vi "Main_Console.vi"(0 "Value_In":string="0" caption="Value In", 5 "Command":T1(ring), 7 "Log_File_Folder":path=path "D:/Assignments/Assignment-4/Assignment-4.1/Assignment-4.1-LV21V/CSV/Logger.csv" caption="Log File Folder", 9 "Stop":bool) -> (4 "Value_Out":string caption="Value Out")   [LabVIEW 2021]
doc: "This VI is the Console VI which communicate with Sour_Meas_instrument."
uses:
  <vilib>/Utility/file.llb/Write Delimited Spreadsheet (string).vi
panel:
  out "Error_Out":errorcluster
  in  "Error_In":errorcluster
  # "Control"
  # "Display"
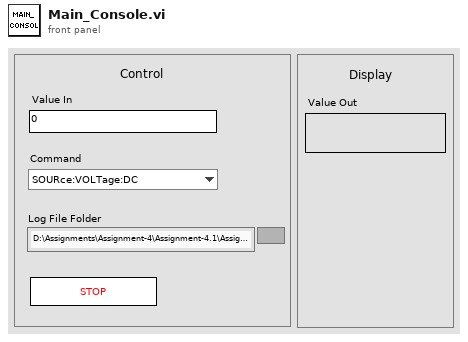
[diagram p1: front panel]
types:
  T1 = enum16{"SOURce:VOLTage:DC", "SOURce:CURRent:DC", "MEASure:VOLTage:DC?", "MEASure:CURRent:DC?"}
  T2 = enum16{"Left Button", "Center Button", "Right Button", "Window Close"}
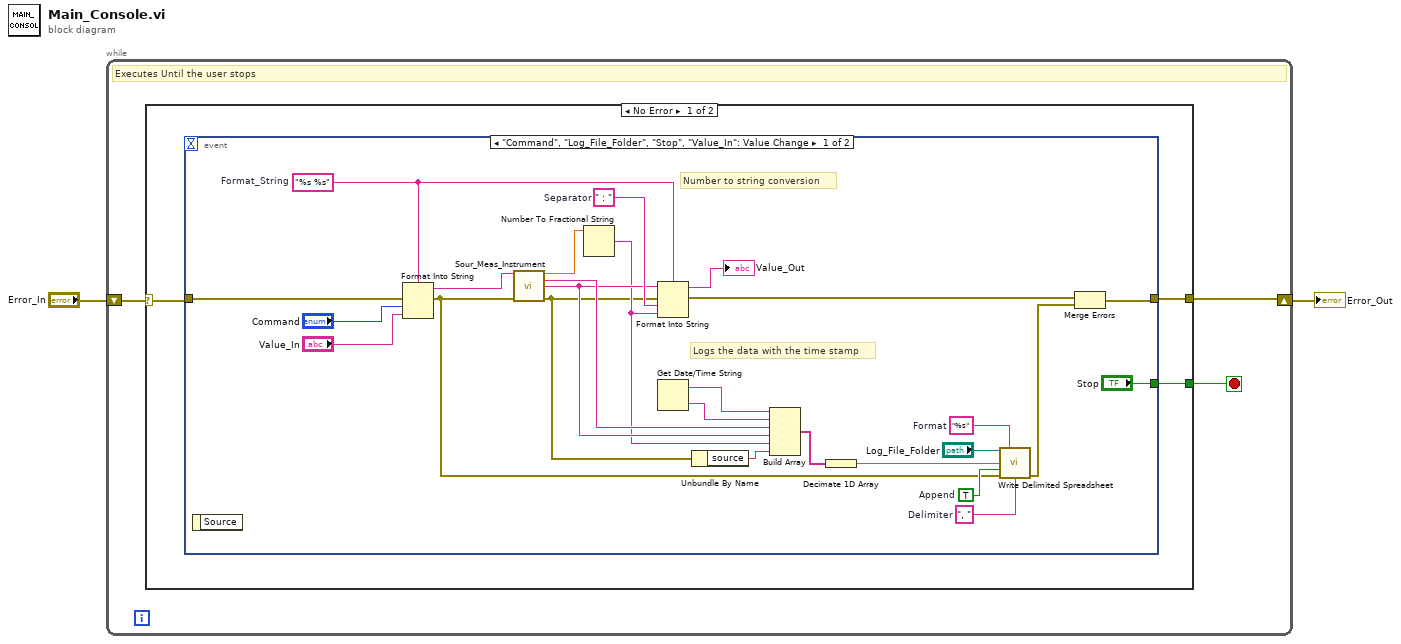
[diagram p0: block diagram]
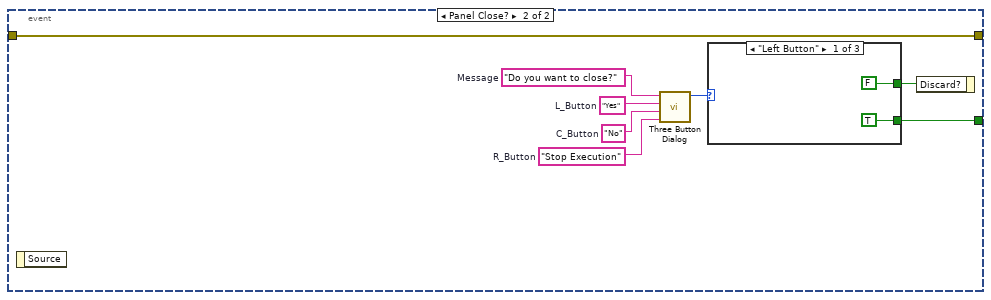
[diagram p2: hidden frame]
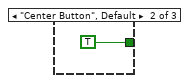
[diagram p3: hidden frame]
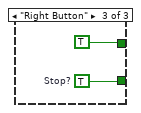
[diagram p4: hidden frame]
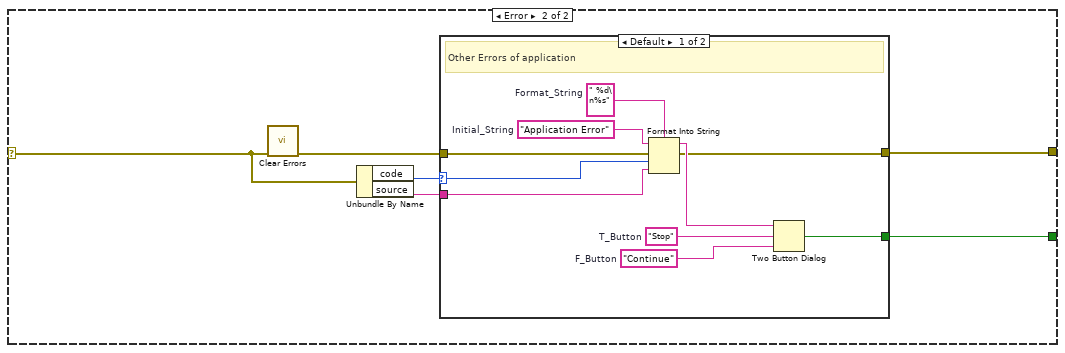
[diagram p5: hidden frame]
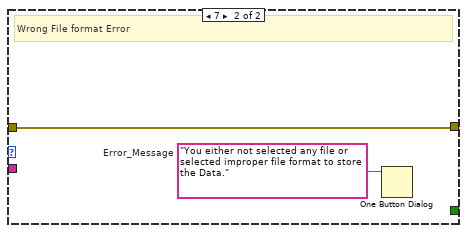
[diagram p6: hidden frame]
diagram:
  n1 = while {
    shift-right: [w3] -> w2
    shift-left: "Error_In" -> [w4]
    stop <- w5 stop-if-true
    # "Executes Until the user stops"
    n2 = case shown="No Error" w4 {
      selector: w4 -> [w7 w53]
      tunnel: [w8 w50] -> w5
      tunnel: [w6 w48] -> w3
      frame No Error {
        n3 = event shown="[0] \"Command\", \"Log_File_Folder\", \"Stop\", \"Value_In\": Value Change" {
          selector: _ -> [_ _]
          dyn-events: _ -> [_ _]
          timeout: _ -> [_ _]
          tunnel: ["Stop" w36] -> w8
          tunnel: w7 -> [w12 w35]
          tunnel: [w11 w35] -> w6
          event "Command", "Log_File_Folder", "Stop", "Value_In": Value Change {
            w26 = TRUE  # Append
            w32 = "%s"  # Format
            w23 = ", "  # Delimiter
            w33 = " : "  # Separator
            w9 = "%s %s"  # Format_String
            # "Number to string conversion"
            # "Logs the data with the time stamp"
            n4 = event-data() -> ()  [unwired: 1 in, 1 out]
            n5 = Format Into String(format string=w9, error in=w12, "Command", "Value_In") -> (resulting string=w14:string, error out=w13:errorcluster)  [unwired: 1 in]
            n6 = call "Sour_Meas_Instrument.vi"("Command"=w14, "Error_In"=w13) -> ("Responce"=w34:dbl, "Action"=w31:string, "Parameter"=w30:string, "Error_Out"=w18:errorcluster)  [unwired: 10 in]
            n7 = Number To Fractional String(number=w34) -> (F-format string=w29:string)  [unwired: 3 in]
            n8 = Format Into String(format string=w9, initial string=w30, error in=w18, w33, w29) -> (resulting string=→"Value_Out":string, error out=w21:errorcluster)
            n9 = Get Date/Time String() -> (date string=w25:string, time string=w24:string)  [unwired: 3 in]
            n10 = Unbundle By Name(w18) -> ("source"=w19:string)
            n11 = Build Array(w25, w24, w31, w30, w29, w19) -> (w28:string[])
            n12 = Decimate 1D Array(w28) -> (w27:string[])
            n13 = call-poly <vilib>:"Write Delimited Spreadsheet.vi"("file path (dialog if empty)"="Log_File_Folder", "format (%s)"=w32, "1D data"=w27, "append to file? (new file:F)"=w26, "error in (no error)"=w13, "delimiter (\\t)"=w23) -> ("error out"=w22:errorcluster)  [unwired: 8 in, 1 out]
            n14 = Merge Errors(w21, w22) -> (w11:errorcluster)
          }
          event Panel Close? {
            w39 = "Stop Execution"  # R_Button
            w40 = "No"  # C_Button
            w41 = "Yes"  # L_Button
            w42 = "Do you want to close?"  # Message
            n15 = event-data() -> ()  [unwired: 1 in, 1 out]
            n16 = call <vilib>:"Three Button Dialog.vi"("Right Button Text (\"Cancel\")"=w39, "Center Button Text (\"No\")"=w40, "Left Button Text (\"Yes\")"=w41, "message"=w42) -> ("Which Button?"=w38:T2)  [unwired: 7 in]
            n17 = case shown="\"Left Button\"" w38 {
              tunnel: [FALSE TRUE TRUE] -> w37
              tunnel: [TRUE _ w47] -> w36
              frame "Left Button" {
              }
              frame "Center Button", Default {
              }
              frame "Right Button" {
                w47 = TRUE  # Stop?
              }
            }
            n18 = event-data ("Event Filter Node")("Discard?"=w37) -> ()  [unwired: 1 in, 1 out]
          }
        }
      }
      frame Error {
        n19 = call <vilib>:"Clear Errors.vi"("error in (no error)"=w53) -> ("error out"=w49:errorcluster)  [unwired: 5 in, 1 out]
        n20 = Unbundle By Name(w53) -> ("code"=w52:i32, "source"=w51:string)
        n21 = case shown="Default" w52 {
          selector: w52 -> [w63 _]
          tunnel: w51 -> [w54 _]
          tunnel: [w59 _] -> w50
          tunnel: w49 -> [w57 w64]
          tunnel: [w56 w64] -> w48
          frame Default {
            w55 = " %d\n%s"  # Format_String
            w58 = "Application Error"  # Initial_String
            w60 = "Stop"  # T_Button
            w61 = "Continue"  # F_Button
            # "Other Errors of application"
            n22 = Format Into String(format string=w55, initial string=w58, error in=w57, w63, w54) -> (resulting string=w62:string, error out=w56:errorcluster)
            n23 = Two Button Dialog(message=w62, 1:w61, 2:w60) -> (T button?=w59:bool)
          }
          frame 7 {
            w65 = "You either not selected any file or selected improper file format to store the Data."  # Error_Message
            # "Wrong File format Error"
            n24 = One Button Dialog(message=w65) -> ()  [unwired: 1 in, 1 out]
          }
        }
      }
    }
  }
  "Error_Out" <- w2
